vi "Acc.vi"() -> ()   [LabVIEW 2020]
panel:
  in  "Lower Cut-Off [Hz]":dbl=2.0 caption="Lower Cut-Off"
  out "Filtered Signal":dynamicdata(graph)
  in  "Recording":bool
  in  "Motor Trottle":dbl(slide) scale=0.0..5.0
  out "Output":dbl
  out "SD AccZ 2":dbl
  out "Acc Y 4":dynamicdata(graph)
  out "SD AccY 2":dbl
  out "Acc Y 3":dynamicdata(graph)
  out "SD AccX 2":dbl
  out "Acc X 2":dynamicdata(graph)
  out "SD AccZ":dbl
  out "Acc Y 2":dynamicdata(graph)
  out "SD AccY":dbl
  out "Acc Y":dynamicdata(graph)
  out "SD AccX":dbl
  out "Acc X":dynamicdata(graph)
  out "Raw Voltage Output":dynamicdata(graph) caption="Raw Voltage Output Dx"
  in  "STOP":bool
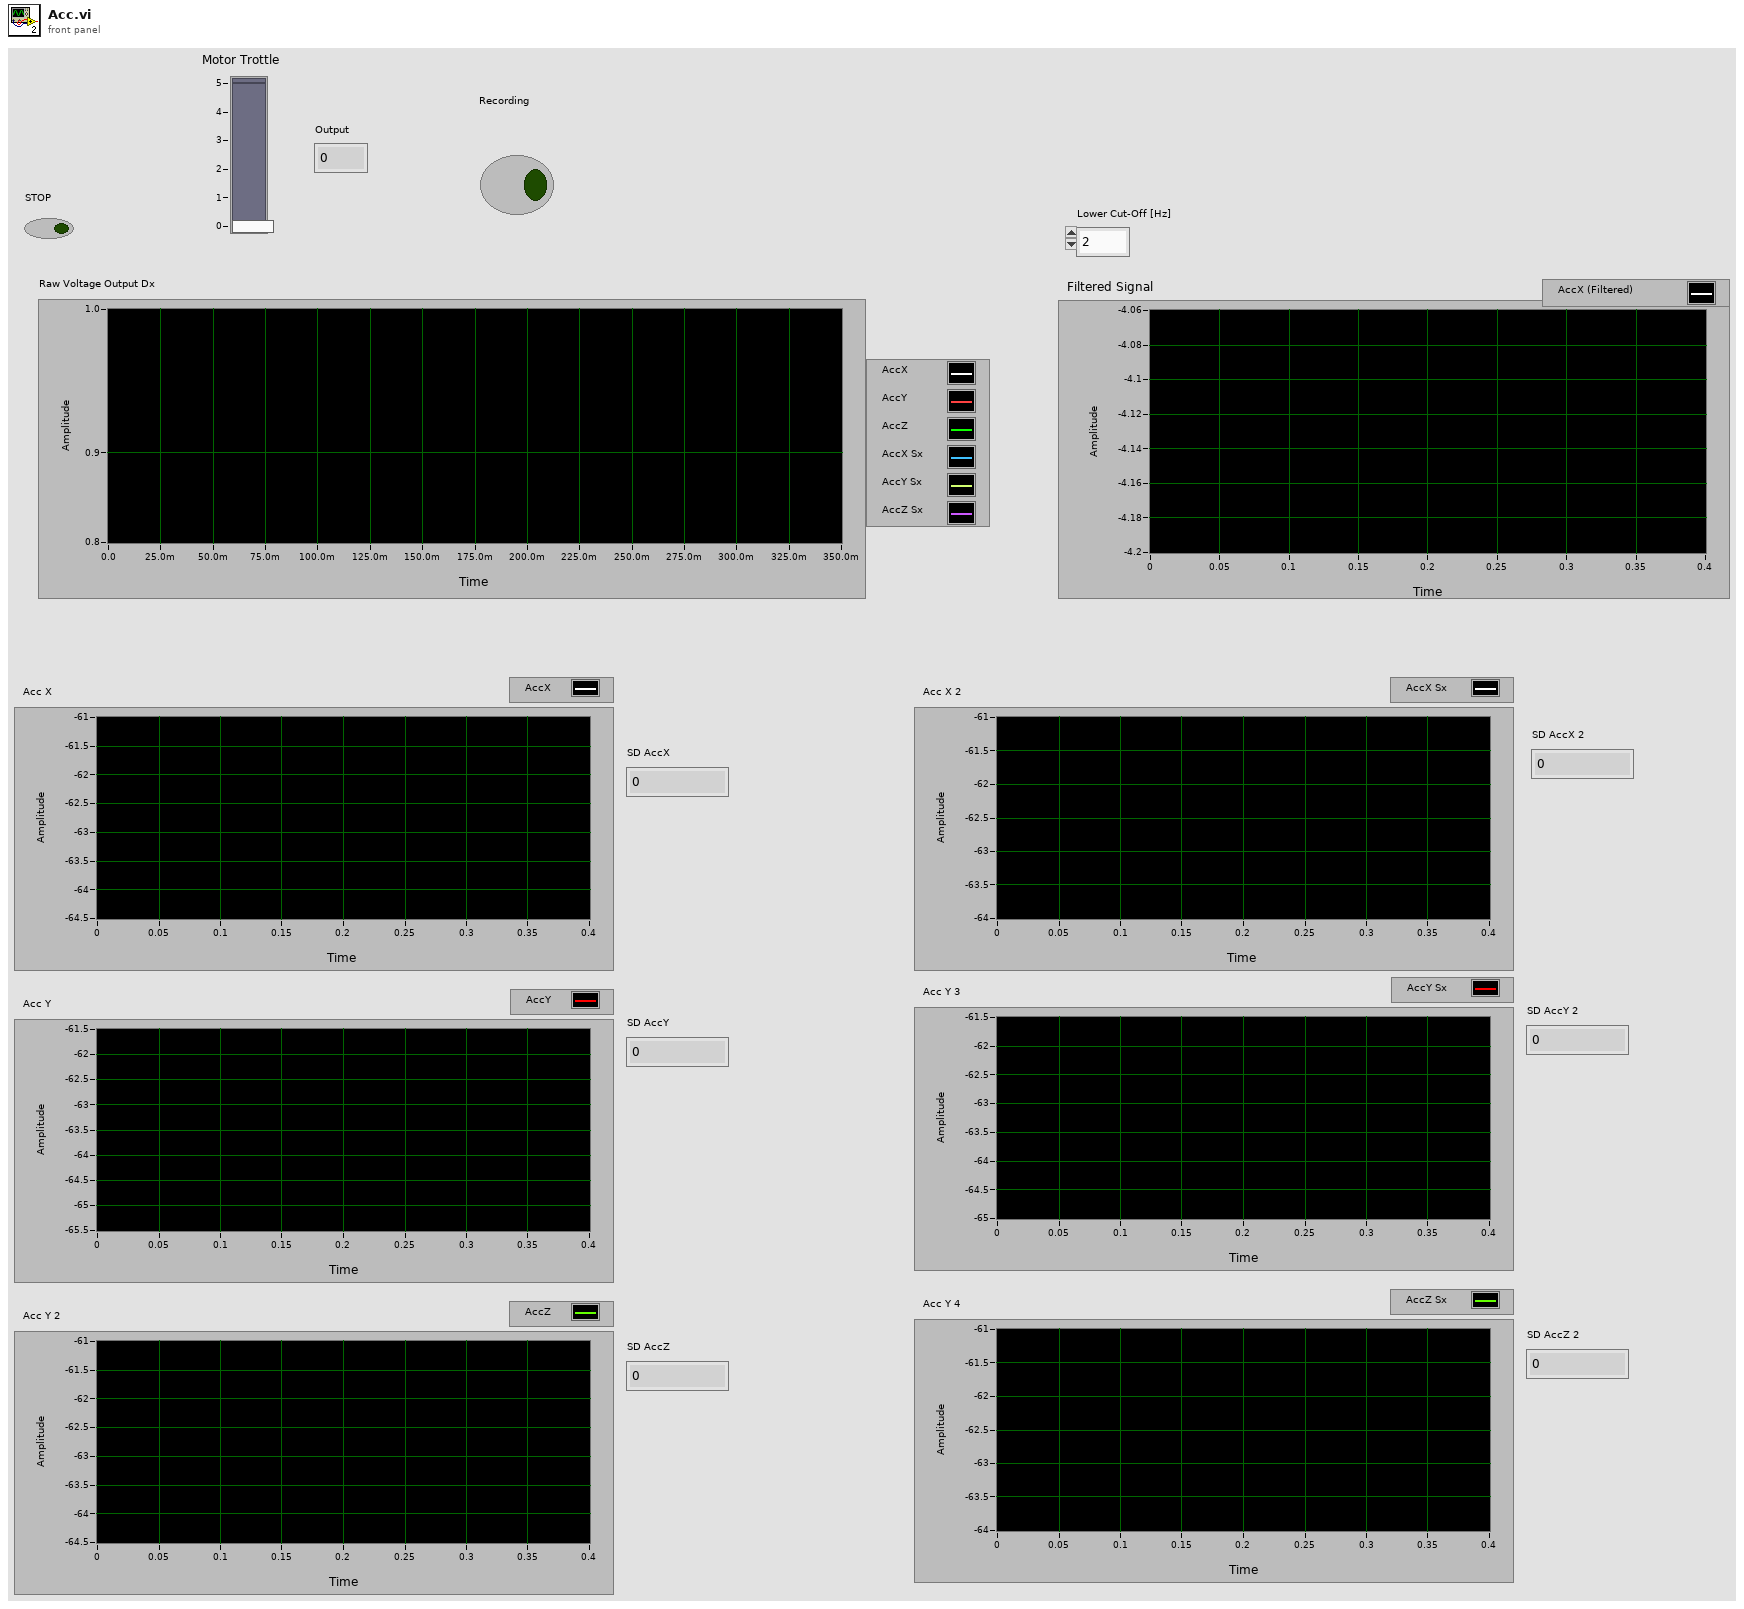
[diagram p1: front panel]
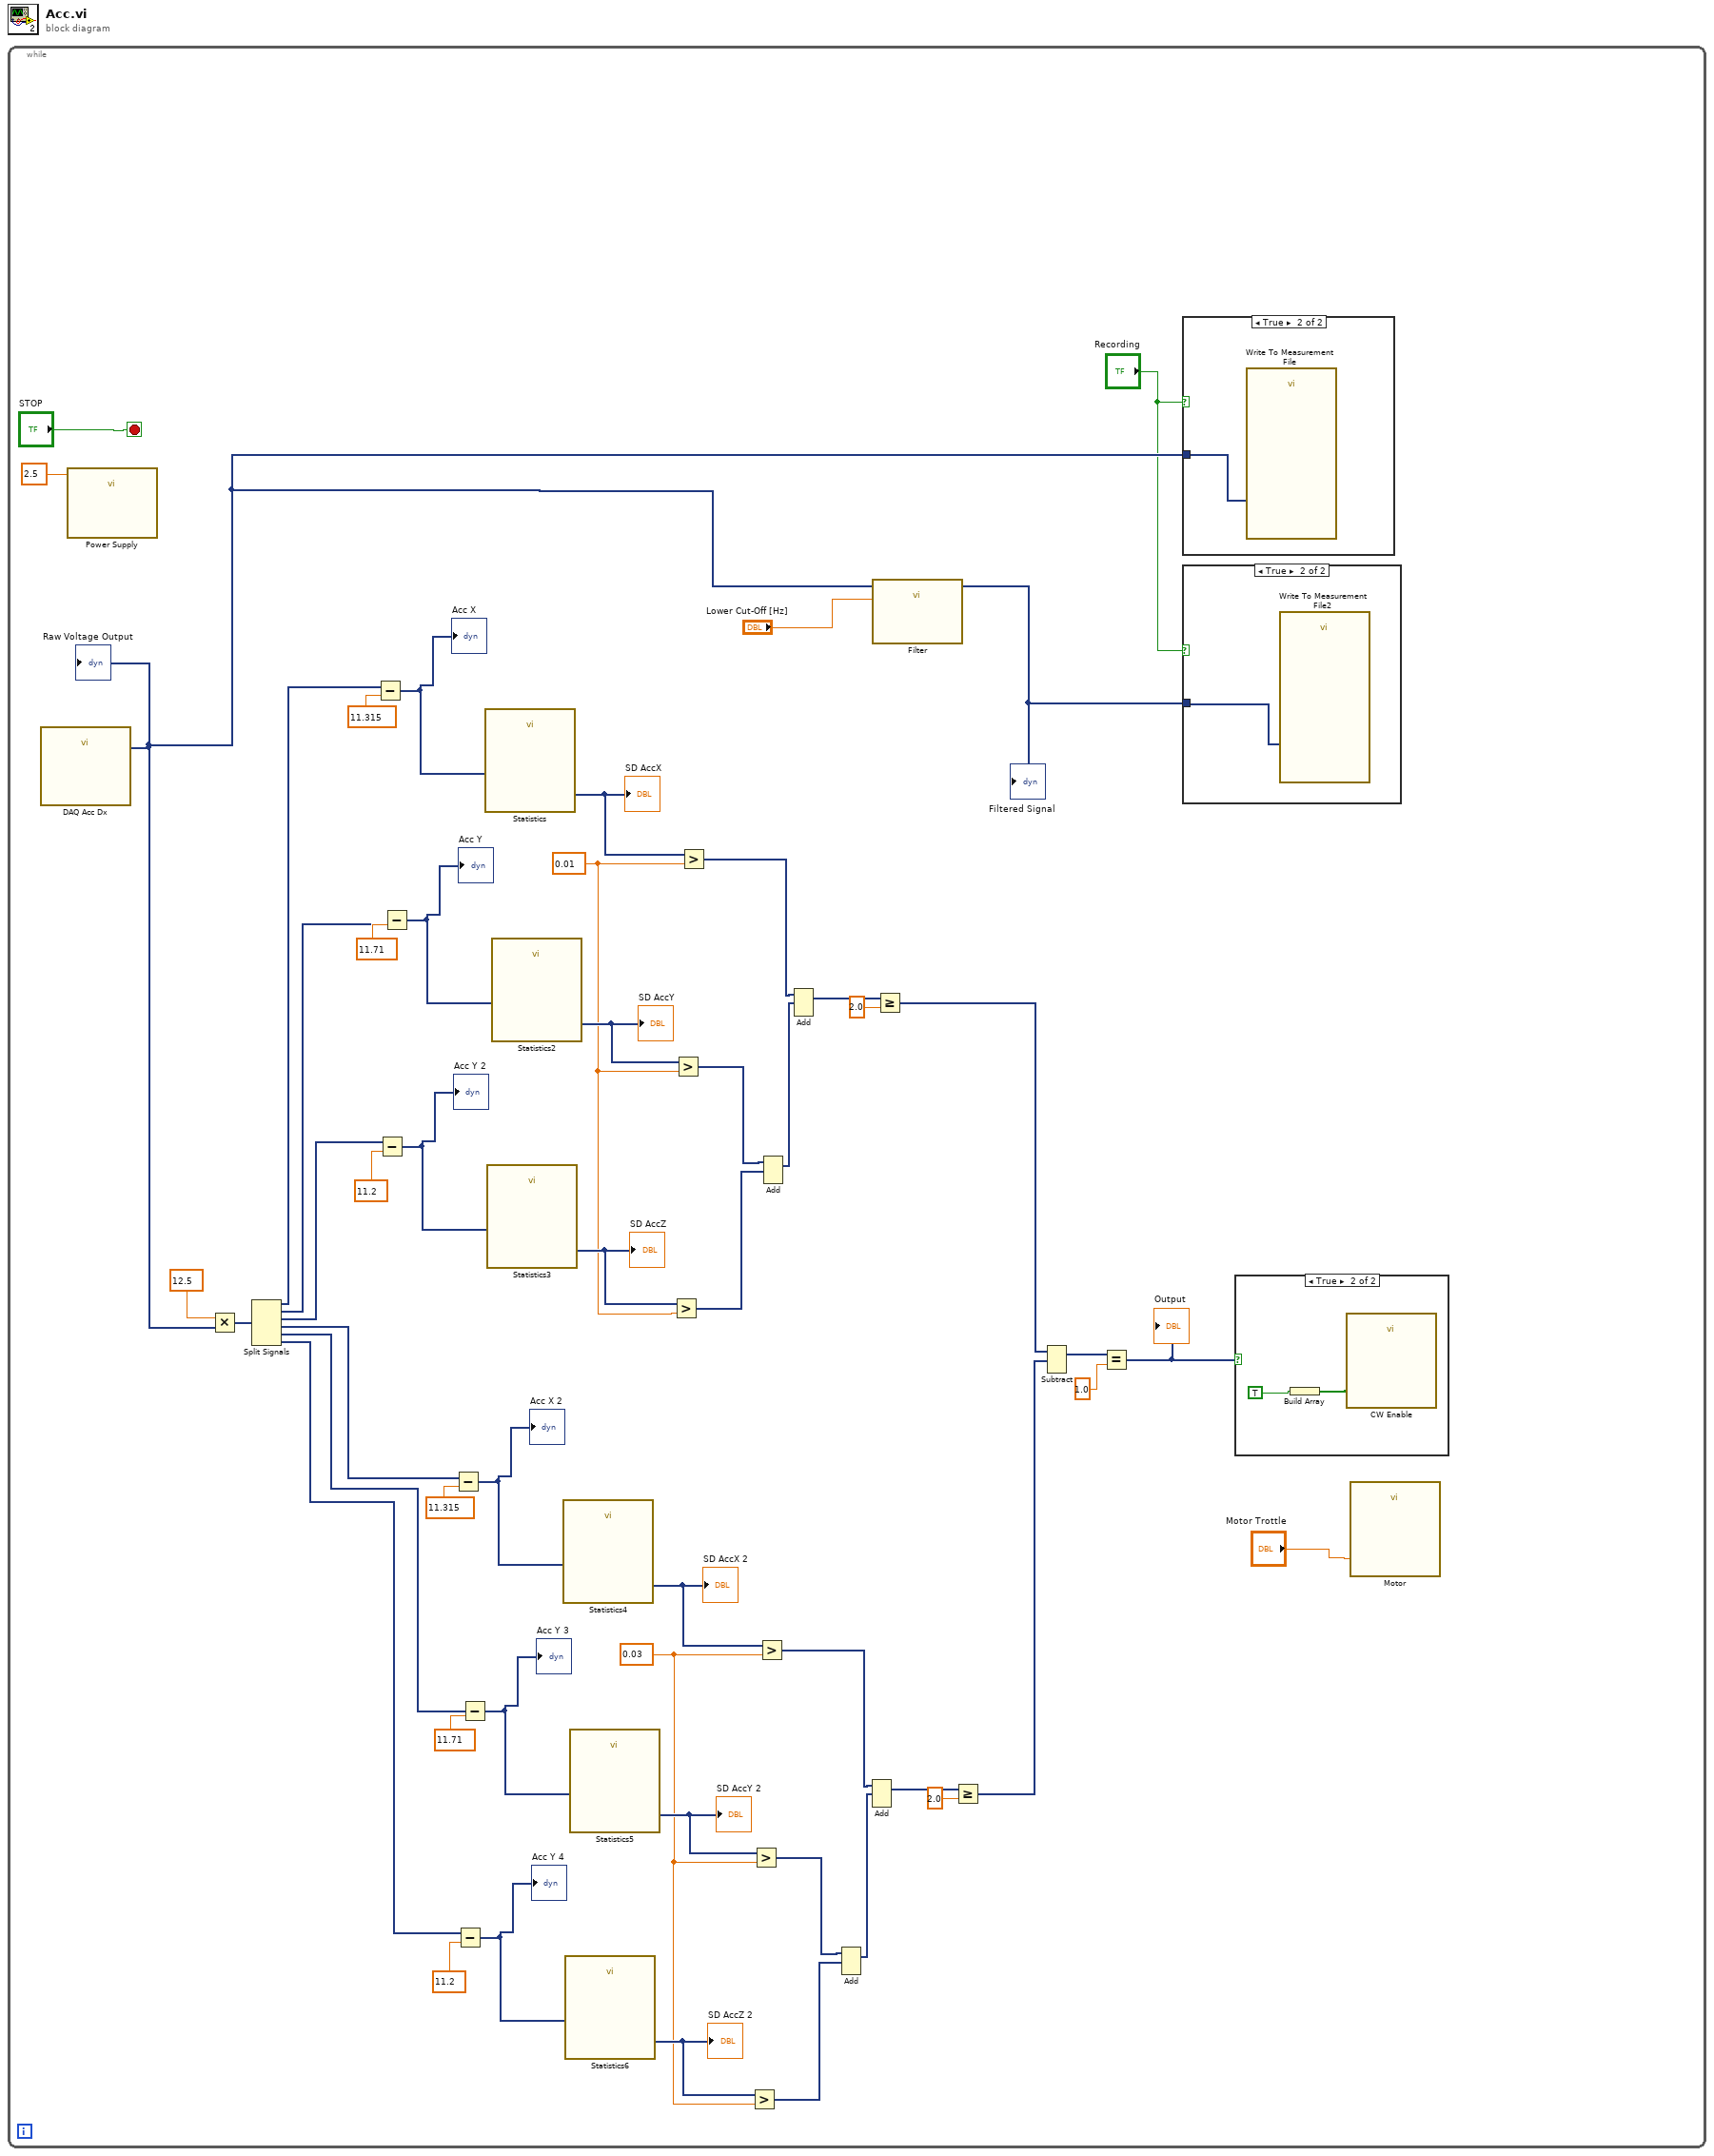
[diagram p0: block diagram]
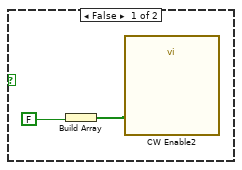
[diagram p4: hidden frame]
diagram:
  n1 = while {
    stop <- "STOP" stop-if-true
    w8 = 0.03 ("y")
    w9 = 0.01 ("y")
    n2 = call "DAQ Acc Dx"() -> ("data"=w3:dynamicdata)  [unwired: 16 in, 3 out]
    "Raw Voltage Output" <- w3
    n3 = call "Power Supply"("data"=2.5) -> ()  [unwired: 17 in, 2 out]
    n4 = Multiply(x=12.5, y=w3) -> (x*y=w5:dynamicdata)
    n5 = Split Signals(w5) -> (w50:dynamicdata, w44:dynamicdata, w42:dynamicdata, w12:dynamicdata, w11:dynamicdata, w10:dynamicdata)  [unwired: 6 in]
    n6 = Subtract(x=w50, y=11.315) -> (x-y=w48:dynamicdata)
    "Acc X" <- w48
    n7 = Subtract(x=w42, y=11.2) -> (x-y=w40:dynamicdata)
    "Acc Y 2" <- w40
    n8 = Subtract(x=w44, y=11.71) -> (x-y=w46:dynamicdata)
    "Acc Y" <- w46
    n9 = Subtract(x=w12, y=11.315) -> (x-y=w31:dynamicdata)
    "Acc X 2" <- w31
    n10 = Subtract(x=w10, y=11.2) -> (x-y=w25:dynamicdata)
    "Acc Y 4" <- w25
    n11 = Subtract(x=w11, y=11.71) -> (x-y=w29:dynamicdata)
    "Acc Y 3" <- w29
    n12 = call "Statistics"("Signals"=w48) -> ("Standard Dev"=w41:dynamicdata)  [unwired: 25 in, 1 out]
    "SD AccX" <- w41
    n13 = call "Statistics3"("Signals"=w40) -> ("Standard Dev"=w38:dynamicdata)  [unwired: 25 in, 1 out]
    "SD AccZ" <- w38
    n14 = call "Statistics2"("Signals"=w46) -> ("Standard Dev"=w39:dynamicdata)  [unwired: 25 in, 1 out]
    "SD AccY" <- w39
    n15 = call "Statistics4"("Signals"=w31) -> ("Standard Dev"=w26:dynamicdata)  [unwired: 25 in, 1 out]
    "SD AccX 2" <- w26
    n16 = call "Statistics6"("Signals"=w25) -> ("Standard Dev"=w23:dynamicdata)  [unwired: 25 in, 1 out]
    "SD AccZ 2" <- w23
    n17 = call "Statistics5"("Signals"=w29) -> ("Standard Dev"=w24:dynamicdata)  [unwired: 25 in, 1 out]
    "SD AccY 2" <- w24
    n18 = Greater?(x=w38, y=w9) -> (0:w37:dynamicdata)
    n19 = Greater?(x=w39, y=w9) -> (0:w36:dynamicdata)
    n20 = Greater?(x=w41, y=w9) -> (0:w34:dynamicdata)
    n21 = Greater?(x=w23, y=w8) -> (0:w22:dynamicdata)
    n22 = Greater?(x=w24, y=w8) -> (0:w21:dynamicdata)
    n23 = Greater?(x=w26, y=w8) -> (0:w19:dynamicdata)
    n24 = Add(1:w37, 2:w36) -> (0:w35:dynamicdata)  [unwired: 1 in, 1 out]
    n25 = Add(1:w35, 2:w34) -> (0:w33:dynamicdata)  [unwired: 1 in, 1 out]
    n26 = Add(1:w22, 2:w21) -> (0:w20:dynamicdata)  [unwired: 1 in, 1 out]
    n27 = Add(1:w20, 2:w19) -> (0:w18:dynamicdata)  [unwired: 1 in, 1 out]
    n28 = call "Filter"("Lower Cut-Off"="Lower Cut-Off [Hz]", "Signal"=w3) -> ("Filtered Signal"=w4:dynamicdata)  [unwired: 8 in, 1 out]
    "Filtered Signal" <- w4
    n29 = Greater Or Equal?(x=w33, y=2.0) -> (x >= y?=w15:dynamicdata)
    n30 = Greater Or Equal?(x=w18, y=2.0) -> (x >= y?=w16:dynamicdata)
    n31 = Subtract(1:w16, 2:w15) -> (0:w13:dynamicdata)  [unwired: 1 in, 1 out]
    n32 = Equal?(x=w13, y=1.0) -> (x = y?=w7:dynamicdata)
    "Output" <- w7
    n33 = case shown="True" "Recording" {
      tunnel: w3 -> [_ w54]
      frame False {
      }
      frame True {
        n34 = call "Write To Measurement File"("Signals"=w54) -> ()  [unwired: 16 in, 3 out]
      }
    }
    n35 = case shown="True" "Recording" {
      tunnel: w4 -> [_ w53]
      frame False {
      }
      frame True {
        n36 = call "Write To Measurement File2"("Signals"=w53) -> ()  [unwired: 16 in, 3 out]
      }
    }
    n37 = case shown="True" w7 {
      frame False {
        n38 = Build Array(FALSE) -> (w56:bool[])
        n39 = call "CW Enable2"("data"=w56) -> ()  [unwired: 17 in, 2 out]
      }
      frame True {
        n40 = Build Array "Build Array"(TRUE) -> (w57:bool[])
        n41 = call "CW Enable"("data"=w57) -> ()  [unwired: 17 in, 2 out]
      }
    }
    n42 = call "Motor"("data"="Motor Trottle") -> ()  [unwired: 17 in, 2 out]
  }
